vi "Test Broadcast Debug Log Filtered by Is Send.vi"(8 "error in (no error)":errorcluster, 11 "Test Case In":refnum<class "Debugger Test.lvclass">) -> (0 "error out":errorcluster, 3 "Test Case Out":refnum<class "Debugger Test.lvclass">)   [LabVIEW 2020, in "Debugger Test.lvclass"]
uses:
  Debugger Test.lvclass
  C:/Program Files (x86)/National Instruments/LabVIEW 2020/vi.lib/Astemes/LUnit/Test Case.lvclass
  source/Debugger/Debugger.lvclass
  C:/Users/anton/Documents/GitHub/triarc-debugger/source/Process/Debug Process.lvclass
  source/Debug Data/Raw Debug Data.ctl
  source/Process/Debug Process.lvclass/Debug Process.ctl
  <vilib>/Astemes/LUnit/Test Case.lvclass/Test Case.ctl
  <vilib>/Astemes/LUnit/LUnit Assertion Result.lvclass/LUnit Assertion Result.ctl
  <vilib>/Astemes/LUnit/LUnit Test Case Result.lvclass/LUnit Test Case Result.ctl
  <vilib>/Astemes/LUnit/LUnit Method Result.lvclass/LUnit Method Result.ctl
  01074fa8-ee8a-411d-bc8b-fc92c4f90959.vi
  source/Process/Public/Lifecycle/Get Lifecycle State.vi
  source/Process/Private/SubVIs/Wait for finish.vi
  source/Process/Protected/Messaging/Enqueue Message.vi
  source/Process/Private/SubVIs/Set Lifecycle State.vi
  <vilib>/Astemes/LUnit/Palette/Pass.vi
  <vilib>/Astemes/LUnit/Palette/Fail.vi
  <vilib>/Astemes/LUnit/Compare Variants.vi
  <vilib>/Astemes/LUnit/Describe Comparison.vi
  <vilib>/Astemes/LUnit/Set Assertion Type.vi
  <vilib>/Utility/error.llb/Clear Errors.vi
  <vilib>/Astemes/LUnit/Add test result.vi
  <vilib>/Astemes/LUnit/LUnit Write Passed.vi
  <vilib>/Astemes/LUnit/LUnit Write Message.vi
  <vilib>/Astemes/LUnit/LUnit Write Description.vi
  <vilib>/Astemes/LUnit/Variant to string.vi
  <vilib>/Astemes/LUnit/LUnit Write Assertion Type.vi
  <vilib>/Astemes/LUnit/LUnit Record Assertion Result.vi
  <vilib>/Astemes/LUnit/LUnit Aggregate Assertion Results.vi
  <vilib>/Astemes/LUnit/Assertion Result/LUnit Read Status.vi
  <vilib>/Astemes/LUnit/LUnit Read Message.vi
  <vilib>/Astemes/LUnit/LUnit Read Description.vi
  <vilib>/Astemes/LUnit/Method Result/LUnit Merge Status.vi
  <vilib>/Astemes/LUnit/LUnit Concatenate result strings.vi
  <vilib>/Utility/error.llb/Error Cluster From Error Code.vi
  <vilib>/Utility/Data Type/Get Type Information.vi
  <vilib>/Utility/LVClass/Get LV Class Name.vi
  <vilib>/Astemes/LUnit/LUnit Assertion Result.lvclass
  source/Process/Debug Process.lvclass
  Debugger Test.lvclass/Debugger Test.ctl
  source/Debug Data/Debug Data.lvclass
  C:/Users/anton/Documents/GitHub/triarc-debugger/source/Debugger/Debugger.lvclass
  C:/Users/anton/Documents/GitHub/triarc-debugger/source/Debug Data Event/Debug Data Listener.lvclass
  <vilib>/Astemes/Triarc Framework/Broadcast Event Helpers/Broadcast Event Helpers.lvlib
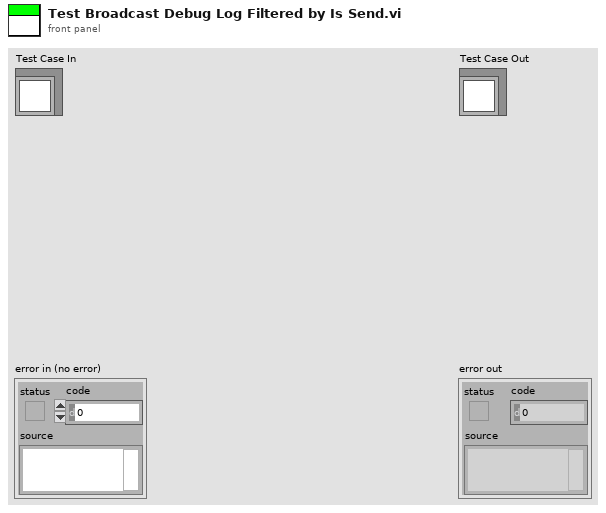
[diagram p1: front panel]
types:
  T1 = typedef "Debug Data.lvclass/Raw Debug Data.ctl" = cluster{"Action":string, "Call Chain":string, "Process":string, "Message":string, "Message Data":variant, "Time":dbl}
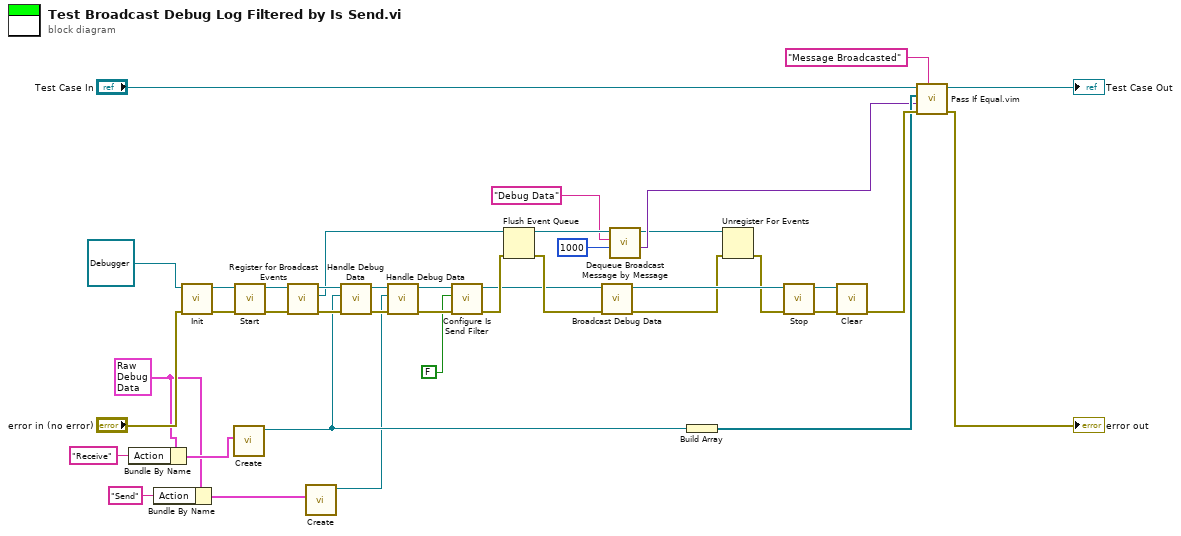
[diagram p0: block diagram]
diagram:
  w12 = T1 {"Action"="", "Call Chain"="", "Process"="", "Message"="", "Message Data"=variant, "Time"=0.0} ("Debug Data Cluster")
  n1 = Bundle By Name(cluster=w12, "Action"="Receive" ("Process")) -> (w20:T1)
  n2 = Bundle By Name(cluster=w12, "Action"="Send" ("Process")) -> (w13:T1)
  n3 = call-dynamic "Init.vi"("error in (no error)"="error in (no error)", "Process In"=refnum<class "Debugger.lvclass"> refnum ("Debug Data Event In 2")) -> ("error out"=w36:errorcluster, "Process Out"=w37:refnum<class "Debugger.lvclass">)  [unwired: 8 in]
  n4 = call "Create.vi"("Debug Data Cluster"=w20) -> ("Debug Data out"=w24:refnum<class "Debug Data.lvclass">)  [unwired: 9 in, 1 out]
  n5 = call "Start.vi"("error in (no error)"=w36, "Process In"=w37) -> ("error out"=w34:errorcluster, "Process Out"=w35:refnum<class "Debugger.lvclass">)  [unwired: 7 in, 1 out]
  n6 = call "Register for Broadcast Events.vi"("error in (no error)"=w34, "Process In"=w35) -> ("error out"=w33:errorcluster, "Event Registration Refnum Out"=w21:refnum<event-registration>, "Process Out"=w29:refnum<class "Debugger.lvclass">)  [unwired: 7 in]
  n7 = call "Create.vi"("Debug Data Cluster"=w13) -> ("Debug Data out"=w15:refnum<class "Debug Data.lvclass">)  [unwired: 9 in, 1 out]
  n8 = call-dynamic "Handle Debug Data.vi"("error in (no error)"=w33, "Debug Data.lvclass"=w24, "Debug Data Event In"=w29) -> ("error out"=w17:errorcluster, "Debug Data Event Out"=w18:refnum<class "Debugger.lvclass">)  [unwired: 7 in]
  n9 = call-dynamic "Handle Debug Data.vi"("error in (no error)"=w17, "Debug Data.lvclass"=w15, "Debug Data Event In"=w18) -> ("error out"=w16:errorcluster, "Debug Data Event Out"=w10:refnum<class "Debugger.lvclass">)  [unwired: 7 in]
  n10 = call "Configure Is Send Filter.vi"("error in (no error)"=w16, "Show Send?"=FALSE, "Debugger In"=w10) -> ("error out"=w11:errorcluster, "Debugger Out"=w9:refnum<class "Debugger.lvclass">)  [unwired: 7 in]
  n11 = Flush Event Queue(0:w21, 3:w11) -> (8:w5:refnum<event-registration>, 11:w22:errorcluster)  [unwired: 4 in, 1 out]
  n12 = call "Broadcast Debug Data.vi"("error in (no error)"=w22, "Debugger in"=w9) -> ("error out"=w8:errorcluster, "Debugger out"=w32:refnum<class "Debugger.lvclass">)  [unwired: 8 in]
  n13 = call <vilib>:"Dequeue Broadcast Message by Message.vi"("Timeout (-1)"=1000, "Message"="Debug Data", "Event Registration Refnum"=w5) -> ("Message Data"=w3:variant, "Event Registration Refnum Out"=w2:refnum<event-registration>)  [unwired: 4 in, 3 out]
  n14 = Build Array(w24) -> (w23:refnum<class "Debug Data.lvclass">[])
  n15 = Unregister For Events(event registration refnum=w2, error in=w8) -> (error out=w7:errorcluster)
  n16 = call "Stop.vi"("error in (no error)"=w7, "Process In"=w32) -> ("error out"=w30:errorcluster, "Process Out"=w31:refnum<class "Debugger.lvclass">)  [unwired: 7 in, 1 out]
  n17 = call-dynamic "Clear.vi"("error in (no error)"=w30, "Process In"=w31) -> ("error out"=w26:errorcluster)  [unwired: 9 in]
  n18 = call "Pass If Equal.vim"("Description"="Message Broadcasted", "error in (no error)"=w26, "Actual"=w3, "Expected"=w23, "LUnit Test Case In"="Test Case In") -> ("error out"=→"error out":errorcluster, "LUnit Test Case Out"=→"Test Case Out":refnum<class "Debugger Test.lvclass">)  [unwired: 5 in]
